vi "XIPIN_AXI_APB_Bridge_3_0.vi"   [LabVIEW 2017]
doc: "AXI APB Bridge connects AXI Matser with APB slaves.\n------------------------------------\n<b>Need License</b> : No\n<b>Interface</b> : AXI4"
uses:
  <vilib>/rvi/XilinxIP/XIPIN_XNode/niFpgaXIPIN.xnode
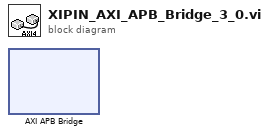
[diagram p0: block diagram]
diagram:
  n1 = xnode ("AXI APB Bridge")() -> ()
